vi "TDMSreaddata.vi"() -> ()   [LabVIEW 2018, in "RW_Protocols.lvlib"]
uses:
  RW_Protocols.lvlib
panel:
  out "Waveform Graph":waveform(dbl)[](graph)
  out "error out":errorcluster
  in  "file path":path=path "D:/Data/Mai/test target/waveformtest.tdms"
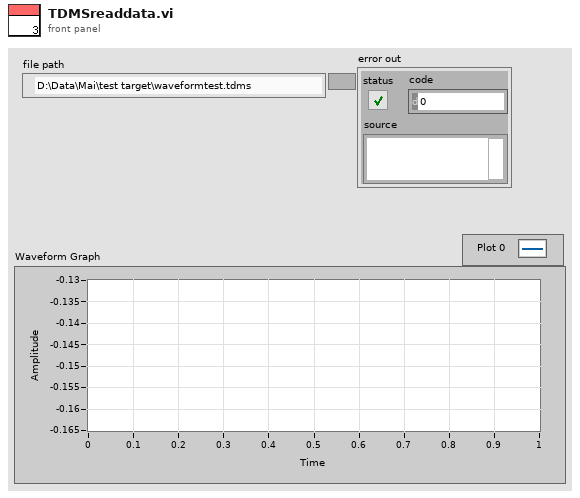
[diagram p1: front panel]
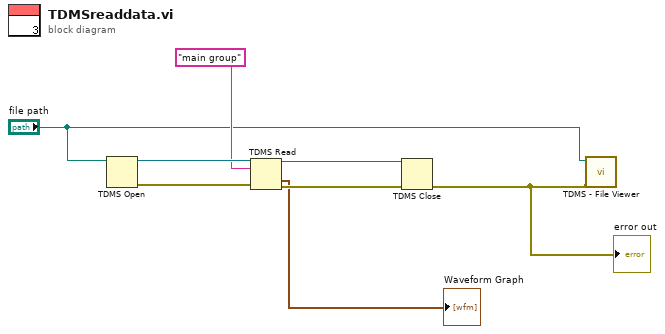
[diagram p0: block diagram]
diagram:
  n1 = TDMS Open(11:"file path") -> (0:w5:errorcluster, 3:w8:refnum<k34>)  [unwired: 6 in]
  n2 = TDMS Read(0:w8, 5:"main group" ("group name in"), 11:w5) -> (4:w7:refnum<k34>, 10:→"Waveform Graph":waveform(dbl)[], 15:w6:errorcluster)  [unwired: 5 in, 3 out]
  n3 = TDMS Close(8:w6, 11:w7) -> (0:w2:errorcluster)  [unwired: 1 out]
  "error out" <- w2
  n4 = call <vilib>:"TDMS - File Viewer.vi"("error in (no error)"=w2, "file path"="file path") -> ()  [unwired: 4 in, 2 out]
